vi "TCE_SaveConfiguration.vi"(0 "input cluster":T1={"Core"={"Current VI Reference"=refnum, "Close Panel on Exit?"=FALSE}, "Image Out"="img_0", "State"=0, "Points"={"Top Left"={"X"=54.0, "Y"=69.0}, "Top Right"={"X"=409.0, "Y"=62.0}, "Bottom Left"={"X"=58.0, "Y"=302.0}, "Bottom Right"={"X"=413.0, "Y"=295.0}, "x space 2"=0.2666666805744171, "y space 2"=15.533334, "x_space"=15.434783, "y_space"=-0.3043478, "Pixels"=array384x21[8064 elements], "Fixpoint"={"X"=460.0, "Y"=26.0}}, "img_array"=["img_0", "img_1", "img_2", "img_3", "img_4", "img_5", "img_6", "img_7", "img_8", "img_9", "img_10", "img_11", "img_12", "img_13", "img_14", "img_15", "img_16", "img_17", "img_18", "img_19", "img_20", "img_21", "img_22", "img_23", "img_24", "img_25", "img_26", "img_27", "img_28", "img_29", "img_30", "img_31", "img_32", "img_33", "img_34", "img_35", "img_36", "img_37", "img_38", "img_39", "img_40", "img_41", "img_42", "img_43", "img_44", "img_45", "img_46", "img_47", "img_48", "img_49", "img_50", "img_51", "img_52", "img_53", "img_54", "img_55", "img_56", "img_57", "img_58", "img_59", "img_60", "img_61", "img_62", "img_63", "img_64", "img_65", "img_66", "img_67", "img_68", "img_69", "img_70", "img_71", "img_72", "img_73", "img_74", "img_75", "img_76", "img_77", "img_78", "img_79", "img_80", "img_81", "img_82", "img_83", "img_84", "img_85", "img_86", "img_87", "img_88", "img_89", "img_90", "img_91", "img_92", "img_93", "img_94", "img_95", "img_96", "img_97", "img_98", "img_99", "img_100", "img_101", "img_102", "img_103", "img_104", "img_105", "img_106", "img_107", "img_108", "img_109", "img_110", "img_111", "img_112", "img_113", "img_114", "img_115", "img_116", "img_117", "img_118", "img_119", "img_120", "img_121", "img_122", "img_123", "img_124", "img_125", "img_126", "img_127", "img_128", "img_129", "img_130", "img_131", "img_132", "img_133", "img_134", "img_135", "img_136", "img_137", "img_138", "img_139", "img_140", "img_141", "img_142", "img_143", "img_144", "img_145", "img_146", "img_147", "img_148", "img_149", "img_150", "img_151", "img_152", "img_153", "img_154", "img_155", "img_156", "img_157", "img_158", "img_159", "img_160", "img_161", "img_162", "img_163", "img_164", "img_165", "img_166", "img_167", "img_168", "img_169", "img_170", "img_171", "img_172", "img_173", "img_174", "img_175", "img_176", "img_177", "img_178", "img_179", "img_180", "img_181", "img_182", "img_183", "img_184", "img_185", "img_186", "img_187", "img_188", "img_189", "img_190", "img_191", "img_192", "img_193", "img_194", "img_195", "img_196", "img_197", "img_198", "img_199", "img_200", "img_201", "img_202", "img_203", "img_204", "img_205", "img_206", "img_207", "img_208", "img_209", "img_210", "img_211", "img_212", "img_213", "img_214", "img_215", "img_216", "img_217", "img_218", "img_219", "img_220", "img_221", "img_222", "img_223", "img_224", "img_225", "img_226", "img_227", "img_228", "img_229", "img_230", "img_231", "img_232", "img_233", "img_234", "img_235", "img_236", "img_237", "img_238", "img_239", "img_240", "img_241", "img_242", "img_243", "img_244", "img_245", "img_246", "img_247", "img_248", "img_249", "img_250", "img_251", "img_252", "img_253"], "Temps"=[], "Temps_Array"=[], "Scan Area"=3.0, "Fixpoint Area"=5.0, "Config"={"Freezing"={"Cutoff"=1.0, "EndIndex"=253}}, "PCR Size"=0, "ImageCount"=253, "ShowGradient"=FALSE} {"Points"."Bottom Right"."Y" format="%.2f"; "Points"."Bottom Right"."X" format="%.2f"; "Points"."Top Left"."Y" format="%.2f"; "Points"."Top Left"."X" format="%.2f"; "Points"."Top Right"."Y" format="%.2f"; "Points"."Top Right"."X" format="%.2f"; "Points"."Bottom Left"."Y" format="%.2f"; "Points"."Bottom Left"."X" format="%.2f"; "Points"."Fixpoint"."Y" format="%.2f"; "Points"."Fixpoint"."X" format="%.2f"}, 1 "Temps":dbl[][](graph)=array384x452[173568 elements], 2 "FreezeTemps":dbl[](array[numeric])=[0.0, 0.0, -9.08812883, 0.0, 0.0, 0.0, 0.0, 0.0, 0.0, 0.0, -9.0747955, -11.51009704, 0.0, 0.0, 0.0, 0.0, 0.0, 0.0, 0.0, 0.0, -6.15635948, 0.0, 0.0, 0.0, 0.0, 0.0, 0.0, -8.47241455, 0.0, 0.0, 0.0, 0.0, -8.26812883, -8.60193836, 0.0, -9.01717645, -9.10955741, -2.30476451, -7.81329159, 0.0, 0.0, -8.8147955, 0.0, 0.0, 0.0, 0.0, 0.0, 0.0, 0.0, 0.0, 0.0, -9.36717645, 0.0, -9.36908121, 0.0, 0.0, 0.0, 0.0, 0.0, -8.96765264, -8.71336693, -8.60431931, 0.0, 0.0, -1.50423713, -1.7488225, -1.82501297, -2.09757047, -2.22863306, -2.2188225, 0.0, -2.1609003, 0.0, -1.86328475, -1.81614189, -1.89328125, -1.82470982, -1.57120345, -1.20787012, -1.03518951, -1.55387115, -1.77453678, -1.94371688, -2.22423713, -2.38757047, -2.36852285, -2.20847878, -2.22471332, -2.0088225, -1.91804315, -1.87381212, -1.93545469, -1.78994791, -1.52739393, -1.45354993, -1.04995142, -1.4709003, -1.6835844, -2.11280856, -2.43614189, -2.38929869, -2.51185618, -2.31705021, -2.47947523, -2.36804666, -2.14804315, -1.88280856, -1.96137999, -1.77053782, -1.76196639, -1.25990735, -1.14233237, 0.0, -1.58757047, -1.94804315, -2.22244258, -2.43709428, -2.38705021, -2.23024468, 0.0, -2.24120345, -2.14376094, -1.79800259, -1.91768067, -1.66929869, -1.65185618, -1.53434734, -1.14328475, -1.20501297, -1.52263202, -1.9575264, -2.0127645, -2.13446292, -2.36709428, -2.51661809, -2.37196639, 0.0, -2.08196639, -2.16865453, -1.73705021, -1.65120345, -1.6962521, -1.4535844, 0.0, -1.21116897, -1.55501297, 0.0, -2.26709428, -2.19786373, -2.44376094, -2.59137999, -2.45025107, -2.16783564, -2.18162766, -2.11285974, -1.98047879, -1.83143117, -1.77815687, -1.49328475, -1.24185268, 0.0, -1.42137999, -1.92137649, -1.96990735, -2.34423713, -2.35518951, -2.38137999, -2.2756657, -2.28484501, -2.3200026, -2.09673946, -1.74995142, -1.61423713, -1.51834631, -1.58769184, 0.0, -1.09960692, -1.67008311, -1.95280856, -2.35280856, -2.19895497, -2.02929869, -1.78263202, -1.86215583, -2.1627645, -2.32423713, -1.99800259, -1.92185618, -1.58787012, -1.45501297, -1.53008311, -1.52640707, 0.0, -1.41280856, -1.84215583, -2.28023365, -2.2609038, -1.86042761, -1.70419307, -2.20995142, -2.3656657, -2.26354993, -2.07019909, -1.83895497, -1.72137999, -1.54133592, -1.51137999, -1.35053782, 0.0, -1.2335844, -1.94137999, -1.8975264, -2.1035844, -2.03167964, -2.15943116, -2.34471332, -2.29990735, -2.12895497, -2.06609783, -1.88596536, -1.86466926, -1.7714902, -1.4775264, -1.26720448, -1.16069278, -1.60190736, -1.88638957, -2.02434734, -2.20126039, -2.29736192, -1.99453678, -2.17905022, -2.21376094, -2.07895497, -2.02817834, -2.07815687, -1.94878802, -1.70072726, -1.31644155, -1.39952641, -1.01640707, -1.33196639, -1.84294025, -2.00389263, -2.13272605, -2.2600026, -2.16627358, -2.23627358, -2.24722596, -2.17722596, -2.15627358, -2.0156657, -1.84021659, -1.70589108, -1.45593088, -1.02232887, 0.0, -1.26947523, -1.78722596, -1.9814902, -2.06177367, -2.32285974, -2.38143117, -2.37638957, -2.32734195, -2.21958544, -2.21436882, -2.06021659, -1.78280506, -1.57804666, -1.47137649, -0.97899904, -0.86054899, -1.07878802, -1.3762521, -1.43800259, -1.76899553, -2.03190736, -2.14831183, -2.02518951, -2.25095498, -1.86596536, -1.95470982, -1.87389263, -1.75829433, -1.53614189, -1.29613839, -1.0053212, 0.0, -1.0400728, -1.33674977, -1.58116897, -1.85129748, -1.9600026, -1.82851934, -2.00115147, -2.20809784, -2.03143117, -1.68310821, -1.57514545, -1.60847878, -1.40995142, -1.40874822, 0.0, -0.92593335, -1.13212383, -0.93518951, -1.84118603, -1.49995142, -1.93578708, -1.8407842, -2.09333593, -1.95783564, -2.05857403, -1.96928127, -2.00268896, -1.82054899, -1.65556332, -1.02674977, -1.34640954, -0.3449387, -0.98508713, -0.93307374, -1.45984993, -1.35714546, -1.50381212, -1.32995142, -1.75023365, -1.58636727, -1.78810625, -1.40042761, -1.8052407, -1.69762165, -1.45878802, -0.87865453, -1.00795467, -0.29116897, -1.1165157, -1.05545469, -1.57763006, -1.12294025, -1.50688326, -1.39067528, -1.25328125, -1.65212204, -1.71883978, -1.69748796, -1.71526146, -1.46428832, -1.38116897, -1.05889755, -1.07318327, -0.27714546, -0.77333593, -0.86878802, -1.24763006, -1.20413474, -0.88768067, -1.12126039, -1.23177367, -1.29413474, -1.30573765, -1.18816803, -1.13190736, -0.72913073, -1.02509752, -0.25804666, -0.07781814, -0.83402612, -1.28878802, -1.82334435, -1.44545469, -1.83603951, -1.15947172, -1.9512785, -1.58047879, -1.42353243, -1.46619308, -1.35994791, -1.64260002, -1.38115147, -1.34531089, -1.4581186, -0.9295966], 3 "MeltTemps":dbl[](array[numeric])=[0.0, 0.0, -0.4342733, 0.0, 0.0, 0.0, 0.0, 0.0, 0.0, 0.0, -0.62680341, -0.51224316, 0.0, 0.0, 0.0, 0.0, 0.0, 0.0, 0.0, 0.0, -0.22420383, 0.0, 0.0, 0.0, 0.0, 0.0, 0.0, -0.49056915, 0.0, 0.0, 0.0, 0.0, -0.43469229, -0.33454438, 0.0, -0.71724972, -0.58354536, 0.3398814, 0.1094774, 0.0, 0.0, -0.21594961, 0.0, 0.0, 0.0, 0.0, 0.0, 0.0, 0.0, 0.0, 0.0, 0.08689311, 0.0, 0.19815221, 0.0, 0.0, 0.0, 0.0, 0.0, 0.21934158, -0.38069337, 0.32423894, 0.0, 0.0, -0.27254066, -0.24847196, -0.2403621, -0.27746832, -0.29275768, -0.38444542, 0.0, -0.31968351, 0.0, -0.28131448, -0.26609101, -0.25751958, -0.17132911, -0.15323387, 0.08177022, -0.18364134, -0.28847196, -0.1565672, -0.20894815, -0.27083829, -0.37940972, -0.35223116, -0.32369543, -0.32889782, -0.28223023, -0.17524899, -0.11682637, -0.14893353, -0.05513863, -0.00223023, -0.01179305, -0.07982523, -0.21275768, -0.09561482, -0.19873113, -0.35111209, -0.39444542, -0.43635018, -0.35635018, -0.38635018, -0.33682637, -0.2253978, -0.17704339, -0.07323387, -0.1050883, -0.08607876, 0.03129403, -0.1065672, 0.0, -0.03799577, -0.14968351, -0.2506221, -0.38349304, -0.39966972, -0.36275768, 0.0, -0.36030142, -0.18942434, -0.14942434, -0.14492161, -0.07179305, -0.03513863, 0.00174506, -0.15371006, -0.10561482, 0.03468434, -0.20842071, -0.22461118, -0.30301685, -0.34798114, -0.34464781, -0.33083829, 0.0, -0.24417162, -0.20321924, -0.12918216, -0.09323387, 0.03205549, 0.06700831, 0.0, -0.09561482, -0.04858474, 0.0, -0.26492161, -0.36746832, -0.38301685, -0.440781, -0.40873113, -0.23635018, -0.23889782, -0.15649529, -0.14432215, -0.11587399, -0.08908405, 0.04967453, -0.18775359, 0.0, 0.09248042, -0.05799577, -0.19751958, -0.30274305, -0.32443162, -0.33226686, -0.31988591, -0.285124, -0.27744767, -0.22459052, -0.10702876, 0.01105185, 0.01152804, 0.05174506, 0.0, 0.15255573, 0.08318743, -0.09037673, -0.30369543, -0.25466244, -0.2018053, -0.13635018, -0.16323387, -0.30704339, -0.30127878, -0.19275768, -0.12777875, 0.01581375, 0.12581375, 0.10555458, -0.08836967, 0.0, 0.11295661, -0.09847196, -0.2530189, -0.26942434, -0.11254066, -0.18444542, -0.29459052, -0.37098881, -0.27080258, -0.20682637, -0.04228149, -0.05704339, 0.06200423, 0.04841172, -0.05268576, 0.0, 0.22093907, -0.04560257, -0.15275768, -0.22322162, -0.23396923, -0.26842071, -0.34206447, -0.32080166, -0.22442026, -0.18799577, -0.09037673, -0.08561482, -0.02037673, 0.07373196, -0.11965835, 0.1401498, 0.16841172, 0.02412601, -0.08444542, -0.11444542, -0.22982862, -0.21349304, -0.1660191, -0.21792386, -0.20349304, -0.12730256, -0.13730256, -0.01682637, 0.05390899, 0.17581375, -0.14323387, 0.14126887, 0.22628994, 0.06031649, 0.00725695, -0.01063589, -0.10887624, -0.15607876, -0.20604068, -0.19492161, -0.10111209, -0.12063589, -0.05199541, 0.03745934, 0.15533756, 0.19570097, -0.00132911, 0.0, 0.28771851, 0.14364982, -0.01158828, -0.05175497, -0.05206447, -0.11730256, -0.14173338, -0.1453978, -0.10275768, -0.09396923, 0.00412601, 0.02962327, 0.18986546, 0.21581375, 0.07087482, 0.30936411, 0.48046529, 0.2598403, 0.08248042, 0.05914708, -0.00396923, -0.07920732, -0.06323387, -0.05920732, -0.0018053, 0.02105185, 0.03446049, 0.09200423, 0.24510355, 0.33200423, 0.18771851, 0.0, 0.56636525, 0.32962327, 0.27698315, 0.14603077, 0.1246022, 0.01820933, 0.05867089, 0.03222125, 0.1046022, 0.07152804, 0.12867089, 0.12438518, 0.32057566, 0.3498403, 0.0, 0.43650696, 0.67317363, 0.44065096, 0.23826662, 0.18189145, 0.19603077, 0.17348313, 0.0746022, 0.20064757, 0.17079268, 0.13064757, 0.15064757, 0.27555458, 0.34793553, 0.55856053, 0.23729265, 0.64507839, 0.82271123, 0.65141767, 0.49454726, 0.44731763, 0.34175885, 0.30364982, 0.29207614, 0.34630219, 0.28586408, 0.27284624, 0.31963552, 0.41555458, 0.50350811, 0.67427481, 0.32126887, 0.90962327, 0.72110218, 0.63207954, 0.5249117, 0.55724232, 0.35588906, 0.39296886, 0.37112716, 0.39364982, 0.35534981, 0.34318743, 0.48317363, 0.56392124, 0.51684144, 0.78126887, 0.44031649, 0.93438518, 0.8598403, 0.76160335, 0.7246022, 0.61996357, 0.6134328, 0.62317363, 0.6101498, 0.59776884, 0.60174506, 0.65237005, 0.74808434, 0.75538882, 0.77603077, 0.9334328, 0.89628994, 0.46919834, 0.46582838, 0.25269744, 0.32868314, 0.35493328, 0.43676613, 0.22793553, 0.35017138, 0.3305879, 0.41079268, 0.29200423, 0.3396379, 0.38106647, 0.59009947, 0.53628994, 0.55200423], 4 "FrozenFraction":dbl[](array[numeric])=[-0.058823529411764705, -0.058823529411764705, 0.7647058823529411, -0.058823529411764705, -0.058823529411764705, -0.058823529411764705, -0.058823529411764705, -0.058823529411764705, -0.058823529411764705, -0.058823529411764705, 0.7058823529411765, 1.0, -0.058823529411764705, -0.058823529411764705, -0.058823529411764705, -0.058823529411764705, -0.058823529411764705, -0.058823529411764705, -0.058823529411764705, -0.058823529411764705, 0.11764705882352941, -0.058823529411764705, -0.058823529411764705, -0.058823529411764705, -0.058823529411764705, -0.058823529411764705, -0.058823529411764705, 0.29411764705882354, -0.058823529411764705, -0.058823529411764705, -0.058823529411764705, -0.058823529411764705, 0.23529411764705882, 0.35294117647058826, -0.058823529411764705, 0.6470588235294118, 0.8235294117647058, 0.058823529411764705, 0.17647058823529413, -0.058823529411764705, -0.058823529411764705, 0.5294117647058824, -0.058823529411764705, -0.058823529411764705, -0.058823529411764705, -0.058823529411764705, -0.058823529411764705, -0.058823529411764705, -0.058823529411764705, -0.058823529411764705, -0.058823529411764705, 0.8823529411764706, -0.058823529411764705, 0.9411764705882353, -0.058823529411764705, -0.058823529411764705, -0.058823529411764705, -0.058823529411764705, -0.058823529411764705, 0.5882352941176471, 0.47058823529411764, 0.4117647058823529, -0.058823529411764705, -0.058823529411764705, 0.14864864864864866, 0.32432432432432434, 0.43243243243243246, 0.6351351351351351, 0.7972972972972973, 0.7432432432432432, -0.013513513513513514, 0.7027027027027027, -0.013513513513513514, 0.44594594594594594, 0.40540540540540543, 0.4864864864864865, 0.4189189189189189, 0.21621621621621623, 0.08108108108108109, 0.013513513513513514, 0.20270270270270271, 0.36486486486486486, 0.5405405405405406, 0.7702702702702703, 0.918918918918919, 0.8783783783783784, 0.7297297297297297, 0.7837837837837838, 0.5945945945945946, 0.5135135135135135, 0.4594594594594595, 0.527027027027027, 0.3783783783783784, 0.17567567567567569, 0.10810810810810811, 0.02702702702702703, 0.13513513513513514, 0.28378378378378377, 0.6486486486486487, 0.9459459459459459, 0.9324324324324325, 0.9864864864864865, 0.8378378378378378, 0.972972972972973, 0.8648648648648649, 0.6891891891891891, 0.47297297297297297, 0.581081081081081, 0.35135135135135137, 0.33783783783783783, 0.0945945945945946, 0.04054054054054054, -0.013513513513513514, 0.22972972972972974, 0.5540540540540541, 0.7567567567567568, 0.9594594594594594, 0.9054054054054054, 0.8108108108108109, -0.013513513513513514, 0.8243243243243243, 0.6756756756756757, 0.3918918918918919, 0.5, 0.2702702702702703, 0.25675675675675674, 0.1891891891891892, 0.05405405405405406, 0.06756756756756757, 0.16216216216216217, 0.5675675675675675, 0.6081081081081081, 0.6621621621621622, 0.8513513513513513, 1.0, 0.8918918918918919, -0.013513513513513514, 0.6216216216216216, 0.7162162162162162, 0.3108108108108108, 0.24324324324324326, 0.2972972972972973, 0.12162162162162163, -0.013513513513513514, 0.02666666666666667, 0.22666666666666666, -0.013333333333333334, 0.8, 0.7333333333333333, 0.9733333333333334, 1.0, 0.9866666666666667, 0.7066666666666667, 0.72, 0.6533333333333333, 0.5466666666666666, 0.37333333333333335, 0.3466666666666667, 0.14666666666666667, 0.05333333333333334, -0.013333333333333334, 0.10666666666666667, 0.48, 0.5333333333333333, 0.8933333333333333, 0.9333333333333333, 0.96, 0.8133333333333334, 0.84, 0.8666666666666667, 0.6266666666666667, 0.32, 0.26666666666666666, 0.17333333333333334, 0.24, -0.013333333333333334, 0.013333333333333334, 0.28, 0.52, 0.92, 0.7466666666666667, 0.5733333333333334, 0.36, 0.4266666666666667, 0.6933333333333334, 0.88, 0.56, 0.49333333333333335, 0.25333333333333335, 0.12, 0.2, 0.18666666666666668, -0.013333333333333334, 0.09333333333333334, 0.4, 0.8266666666666667, 0.7733333333333333, 0.41333333333333333, 0.29333333333333333, 0.76, 0.9466666666666667, 0.7866666666666666, 0.6133333333333333, 0.38666666666666666, 0.30666666666666664, 0.21333333333333335, 0.16, 0.08, -0.013333333333333334, 0.04, 0.5066666666666667, 0.4666666666666667, 0.64, 0.5866666666666667, 0.68, 0.9066666666666666, 0.8533333333333334, 0.6666666666666666, 0.6, 0.4533333333333333, 0.44, 0.3333333333333333, 0.13333333333333333, 0.06666666666666667, 0.1038961038961039, 0.3246753246753247, 0.5194805194805194, 0.6363636363636364, 0.8311688311688312, 0.948051948051948, 0.5844155844155844, 0.8181818181818182, 0.8571428571428571, 0.7402597402597403, 0.6623376623376623, 0.7272727272727273, 0.5324675324675324, 0.36363636363636365, 0.14285714285714285, 0.19480519480519481, 0.05194805194805195, 0.15584415584415584, 0.4675324675324675, 0.6103896103896104, 0.7532467532467533, 0.935064935064935, 0.7922077922077922, 0.8961038961038961, 0.9090909090909091, 0.8051948051948052, 0.7792207792207793, 0.6233766233766234, 0.45454545454545453, 0.37662337662337664, 0.24675324675324675, 0.06493506493506493, -0.012987012987012988, 0.11688311688311688, 0.42857142857142855, 0.5714285714285714, 0.7142857142857143, 0.961038961038961, 1.0, 0.987012987012987, 0.974025974025974, 0.8831168831168831, 0.8701298701298701, 0.7012987012987013, 0.4155844155844156, 0.2987012987012987, 0.2597402597402597, 0.025974025974025976, 0.012987012987012988, 0.09090909090909091, 0.18181818181818182, 0.23376623376623376, 0.4025974025974026, 0.6883116883116883, 0.7662337662337663, 0.6493506493506493, 0.922077922077922, 0.4935064935064935, 0.5454545454545454, 0.5064935064935064, 0.38961038961038963, 0.2727272727272727, 0.12987012987012986, 0.03896103896103896, -0.012987012987012988, 0.07792207792207792, 0.16883116883116883, 0.3116883116883117, 0.4805194805194805, 0.5584415584415584, 0.44155844155844154, 0.5974025974025974, 0.8441558441558441, 0.6753246753246753, 0.35064935064935066, 0.2857142857142857, 0.33766233766233766, 0.22077922077922077, 0.2077922077922078, -0.012987012987012988, 0.15, 0.3375, 0.1875, 0.9125, 0.6625, 0.925, 0.9, 1.0, 0.95, 0.9875, 0.9625, 0.975, 0.8625, 0.7625, 0.2375, 0.4875, 0.0625, 0.2, 0.175, 0.625, 0.5, 0.675, 0.4625, 0.825, 0.725, 0.8375, 0.5625, 0.85, 0.7875, 0.6125, 0.125, 0.2125, 0.05, 0.2875, 0.25, 0.7, 0.3125, 0.6875, 0.55, 0.4125, 0.75, 0.8125, 0.775, 0.8, 0.6375, 0.5375, 0.2625, 0.275, 0.0375, 0.0875, 0.1125, 0.4, 0.375, 0.1375, 0.3, 0.3875, 0.4375, 0.45, 0.3625, 0.325, 0.075, 0.225, 0.025, 0.0125, 0.1, 0.425, 0.875, 0.5875, 0.8875, 0.35, 0.9375, 0.7125, 0.575, 0.65, 0.5125, 0.7375, 0.525, 0.475, 0.6, 0.1625], 5 "PartitionArray":string[](array[string])=["A, MQ filtered", "A, MQ filtered", "A, MQ filtered", "A, MQ filtered", "A, MQ filtered", "A, MQ filtered", "A, MQ filtered", "A, MQ filtered", "A, MQ filtered", "A, MQ filtered", "A, MQ filtered", "A, MQ filtered", "A, MQ filtered", "A, MQ filtered", "A, MQ filtered", "A, MQ filtered", "A, MQ filtered", "A, MQ filtered", "A, MQ filtered", "A, MQ filtered", "A, MQ filtered", "A, MQ filtered", "A, MQ filtered", "A, MQ filtered", "A, MQ filtered", "A, MQ filtered", "A, MQ filtered", "A, MQ filtered", "A, MQ filtered", "A, MQ filtered", "A, MQ filtered", "A, MQ filtered", "A, MQ filtered", "A, MQ filtered", "A, MQ filtered", "A, MQ filtered", "A, MQ filtered", "A, MQ filtered", "A, MQ filtered", "A, MQ filtered", "A, MQ filtered", "A, MQ filtered", "A, MQ filtered", "A, MQ filtered", "A, MQ filtered", "A, MQ filtered", "A, MQ filtered", "A, MQ filtered", "A, MQ filtered", "A, MQ filtered", "A, MQ filtered", "A, MQ filtered", "A, MQ filtered", "A, MQ filtered", "A, MQ filtered", "A, MQ filtered", "A, MQ filtered", "A, MQ filtered", "A, MQ filtered", "A, MQ filtered", "A, MQ filtered", "A, MQ filtered", "A, MQ filtered", "A, MQ filtered", "B, 220628_Psyringae_L_8days_c1", "B, 220628_Psyringae_L_8days_c1", "B, 220628_Psyringae_L_8days_c1", "B, 220628_Psyringae_L_8days_c1", "B, 220628_Psyringae_L_8days_c1", "B, 220628_Psyringae_L_8days_c1", "B, 220628_Psyringae_L_8days_c1", "B, 220628_Psyringae_L_8days_c1", "B, 220628_Psyringae_L_8days_c1", "B, 220628_Psyringae_L_8days_c1", "B, 220628_Psyringae_L_8days_c1", "B, 220628_Psyringae_L_8days_c1", "B, 220628_Psyringae_L_8days_c1", "B, 220628_Psyringae_L_8days_c1", "B, 220628_Psyringae_L_8days_c1", "B, 220628_Psyringae_L_8days_c1", "B, 220628_Psyringae_L_8days_c1", "B, 220628_Psyringae_L_8days_c1", "B, 220628_Psyringae_L_8days_c1", "B, 220628_Psyringae_L_8days_c1", "B, 220628_Psyringae_L_8days_c1", "B, 220628_Psyringae_L_8days_c1", "B, 220628_Psyringae_L_8days_c1", "B, 220628_Psyringae_L_8days_c1", "B, 220628_Psyringae_L_8days_c1", "B, 220628_Psyringae_L_8days_c1", "B, 220628_Psyringae_L_8days_c1", "B, 220628_Psyringae_L_8days_c1", "B, 220628_Psyringae_L_8days_c1", "B, 220628_Psyringae_L_8days_c1", "B, 220628_Psyringae_L_8days_c1", "B, 220628_Psyringae_L_8days_c1", "B, 220628_Psyringae_L_8days_c1", "B, 220628_Psyringae_L_8days_c1", "B, 220628_Psyringae_L_8days_c1", "B, 220628_Psyringae_L_8days_c1", "B, 220628_Psyringae_L_8days_c1", "B, 220628_Psyringae_L_8days_c1", "B, 220628_Psyringae_L_8days_c1", "B, 220628_Psyringae_L_8days_c1", "B, 220628_Psyringae_L_8days_c1", "B, 220628_Psyringae_L_8days_c1", "B, 220628_Psyringae_L_8days_c1", "B, 220628_Psyringae_L_8days_c1", "B, 220628_Psyringae_L_8days_c1", "B, 220628_Psyringae_L_8days_c1", "B, 220628_Psyringae_L_8days_c1", "B, 220628_Psyringae_L_8days_c1", "B, 220628_Psyringae_L_8days_c1", "B, 220628_Psyringae_L_8days_c1", "B, 220628_Psyringae_L_8days_c1", "B, 220628_Psyringae_L_8days_c1", "B, 220628_Psyringae_L_8days_c1", "B, 220628_Psyringae_L_8days_c1", "B, 220628_Psyringae_L_8days_c1", "B, 220628_Psyringae_L_8days_c1", "B, 220628_Psyringae_L_8days_c1", "B, 220628_Psyringae_L_8days_c1", "B, 220628_Psyringae_L_8days_c1", "B, 220628_Psyringae_L_8days_c1", "B, 220628_Psyringae_L_8days_c1", "B, 220628_Psyringae_L_8days_c1", "B, 220628_Psyringae_L_8days_c1", "B, 220628_Psyringae_L_8days_c1", "B, 220628_Psyringae_L_8days_c1", "B, 220628_Psyringae_L_8days_c1", "B, 220628_Psyringae_L_8days_c1", "B, 220628_Psyringae_L_8days_c1", "B, 220628_Psyringae_L_8days_c1", "B, 220628_Psyringae_L_8days_c1", "B, 220628_Psyringae_L_8days_c1", "B, 220628_Psyringae_L_8days_c1", "B, 220628_Psyringae_L_8days_c1", "B, 220628_Psyringae_L_8days_c1", "B, 220628_Psyringae_L_8days_c1", "B, 220628_Psyringae_L_8days_c1", "B, 220628_Psyringae_L_8days_c1", "B, 220628_Psyringae_L_8days_c1", "B, 220628_Psyringae_L_8days_c1", "B, 220628_Psyringae_L_8days_c1", "C, 220628_Psyringae_L_8days_c1_10fold_dil", "C, 220628_Psyringae_L_8days_c1_10fold_dil", "C, 220628_Psyringae_L_8days_c1_10fold_dil", "C, 220628_Psyringae_L_8days_c1_10fold_dil", "C, 220628_Psyringae_L_8days_c1_10fold_dil", "C, 220628_Psyringae_L_8days_c1_10fold_dil", "C, 220628_Psyringae_L_8days_c1_10fold_dil", "C, 220628_Psyringae_L_8days_c1_10fold_dil", "C, 220628_Psyringae_L_8days_c1_10fold_dil", "C, 220628_Psyringae_L_8days_c1_10fold_dil", "C, 220628_Psyringae_L_8days_c1_10fold_dil", "C, 220628_Psyringae_L_8days_c1_10fold_dil", "C, 220628_Psyringae_L_8days_c1_10fold_dil", "C, 220628_Psyringae_L_8days_c1_10fold_dil", "C, 220628_Psyringae_L_8days_c1_10fold_dil", "C, 220628_Psyringae_L_8days_c1_10fold_dil", "C, 220628_Psyringae_L_8days_c1_10fold_dil", "C, 220628_Psyringae_L_8days_c1_10fold_dil", "C, 220628_Psyringae_L_8days_c1_10fold_dil", "C, 220628_Psyringae_L_8days_c1_10fold_dil", "C, 220628_Psyringae_L_8days_c1_10fold_dil", "C, 220628_Psyringae_L_8days_c1_10fold_dil", "C, 220628_Psyringae_L_8days_c1_10fold_dil", "C, 220628_Psyringae_L_8days_c1_10fold_dil", "C, 220628_Psyringae_L_8days_c1_10fold_dil", "C, 220628_Psyringae_L_8days_c1_10fold_dil", "C, 220628_Psyringae_L_8days_c1_10fold_dil", "C, 220628_Psyringae_L_8days_c1_10fold_dil", "C, 220628_Psyringae_L_8days_c1_10fold_dil", "C, 220628_Psyringae_L_8days_c1_10fold_dil", "C, 220628_Psyringae_L_8days_c1_10fold_dil", "C, 220628_Psyringae_L_8days_c1_10fold_dil", "C, 220628_Psyringae_L_8days_c1_10fold_dil", "C, 220628_Psyringae_L_8days_c1_10fold_dil", "C, 220628_Psyringae_L_8days_c1_10fold_dil", "C, 220628_Psyringae_L_8days_c1_10fold_dil", "C, 220628_Psyringae_L_8days_c1_10fold_dil", "C, 220628_Psyringae_L_8days_c1_10fold_dil", "C, 220628_Psyringae_L_8days_c1_10fold_dil", "C, 220628_Psyringae_L_8days_c1_10fold_dil", "C, 220628_Psyringae_L_8days_c1_10fold_dil", "C, 220628_Psyringae_L_8days_c1_10fold_dil", "C, 220628_Psyringae_L_8days_c1_10fold_dil", "C, 220628_Psyringae_L_8days_c1_10fold_dil", "C, 220628_Psyringae_L_8days_c1_10fold_dil", "C, 220628_Psyringae_L_8days_c1_10fold_dil", "C, 220628_Psyringae_L_8days_c1_10fold_dil", "C, 220628_Psyringae_L_8days_c1_10fold_dil", "C, 220628_Psyringae_L_8days_c1_10fold_dil", "C, 220628_Psyringae_L_8days_c1_10fold_dil", "C, 220628_Psyringae_L_8days_c1_10fold_dil", "C, 220628_Psyringae_L_8days_c1_10fold_dil", "C, 220628_Psyringae_L_8days_c1_10fold_dil", "C, 220628_Psyringae_L_8days_c1_10fold_dil", "C, 220628_Psyringae_L_8days_c1_10fold_dil", "C, 220628_Psyringae_L_8days_c1_10fold_dil", "C, 220628_Psyringae_L_8days_c1_10fold_dil", "C, 220628_Psyringae_L_8days_c1_10fold_dil", "C, 220628_Psyringae_L_8days_c1_10fold_dil", "C, 220628_Psyringae_L_8days_c1_10fold_dil", "C, 220628_Psyringae_L_8days_c1_10fold_dil", "C, 220628_Psyringae_L_8days_c1_10fold_dil", "C, 220628_Psyringae_L_8days_c1_10fold_dil", "C, 220628_Psyringae_L_8days_c1_10fold_dil", "C, 220628_Psyringae_L_8days_c1_10fold_dil", "C, 220628_Psyringae_L_8days_c1_10fold_dil", "C, 220628_Psyringae_L_8days_c1_10fold_dil", "C, 220628_Psyringae_L_8days_c1_10fold_dil", "C, 220628_Psyringae_L_8days_c1_10fold_dil", "C, 220628_Psyringae_L_8days_c1_10fold_dil", "C, 220628_Psyringae_L_8days_c1_10fold_dil", "C, 220628_Psyringae_L_8days_c1_10fold_dil", "C, 220628_Psyringae_L_8days_c1_10fold_dil", "C, 220628_Psyringae_L_8days_c1_10fold_dil", "C, 220628_Psyringae_L_8days_c1_10fold_dil", "C, 220628_Psyringae_L_8days_c1_10fold_dil", "C, 220628_Psyringae_L_8days_c1_10fold_dil", "C, 220628_Psyringae_L_8days_c1_10fold_dil", "C, 220628_Psyringae_L_8days_c1_10fold_dil", "C, 220628_Psyringae_L_8days_c1_10fold_dil", "D, 220628_Psyringae_L_8days_c1_100fold_dil", "D, 220628_Psyringae_L_8days_c1_100fold_dil", "D, 220628_Psyringae_L_8days_c1_100fold_dil", "D, 220628_Psyringae_L_8days_c1_100fold_dil", "D, 220628_Psyringae_L_8days_c1_100fold_dil", "D, 220628_Psyringae_L_8days_c1_100fold_dil", "D, 220628_Psyringae_L_8days_c1_100fold_dil", "D, 220628_Psyringae_L_8days_c1_100fold_dil", "D, 220628_Psyringae_L_8days_c1_100fold_dil", "D, 220628_Psyringae_L_8days_c1_100fold_dil", "D, 220628_Psyringae_L_8days_c1_100fold_dil", "D, 220628_Psyringae_L_8days_c1_100fold_dil", "D, 220628_Psyringae_L_8days_c1_100fold_dil", "D, 220628_Psyringae_L_8days_c1_100fold_dil", "D, 220628_Psyringae_L_8days_c1_100fold_dil", "D, 220628_Psyringae_L_8days_c1_100fold_dil", "D, 220628_Psyringae_L_8days_c1_100fold_dil", "D, 220628_Psyringae_L_8days_c1_100fold_dil", "D, 220628_Psyringae_L_8days_c1_100fold_dil", "D, 220628_Psyringae_L_8days_c1_100fold_dil", "D, 220628_Psyringae_L_8days_c1_100fold_dil", "D, 220628_Psyringae_L_8days_c1_100fold_dil", "D, 220628_Psyringae_L_8days_c1_100fold_dil", "D, 220628_Psyringae_L_8days_c1_100fold_dil", "D, 220628_Psyringae_L_8days_c1_100fold_dil", "D, 220628_Psyringae_L_8days_c1_100fold_dil", "D, 220628_Psyringae_L_8days_c1_100fold_dil", "D, 220628_Psyringae_L_8days_c1_100fold_dil", "D, 220628_Psyringae_L_8days_c1_100fold_dil", "D, 220628_Psyringae_L_8days_c1_100fold_dil", "D, 220628_Psyringae_L_8days_c1_100fold_dil", "D, 220628_Psyringae_L_8days_c1_100fold_dil", "D, 220628_Psyringae_L_8days_c1_100fold_dil", "D, 220628_Psyringae_L_8days_c1_100fold_dil", "D, 220628_Psyringae_L_8days_c1_100fold_dil", "D, 220628_Psyringae_L_8days_c1_100fold_dil", "D, 220628_Psyringae_L_8days_c1_100fold_dil", "D, 220628_Psyringae_L_8days_c1_100fold_dil", "D, 220628_Psyringae_L_8days_c1_100fold_dil", "D, 220628_Psyringae_L_8days_c1_100fold_dil", "D, 220628_Psyringae_L_8days_c1_100fold_dil", "D, 220628_Psyringae_L_8days_c1_100fold_dil", "D, 220628_Psyringae_L_8days_c1_100fold_dil", "D, 220628_Psyringae_L_8days_c1_100fold_dil", "D, 220628_Psyringae_L_8days_c1_100fold_dil", "D, 220628_Psyringae_L_8days_c1_100fold_dil", "D, 220628_Psyringae_L_8days_c1_100fold_dil", "D, 220628_Psyringae_L_8days_c1_100fold_dil", "D, 220628_Psyringae_L_8days_c1_100fold_dil", "D, 220628_Psyringae_L_8days_c1_100fold_dil", "D, 220628_Psyringae_L_8days_c1_100fold_dil", "D, 220628_Psyringae_L_8days_c1_100fold_dil", "D, 220628_Psyringae_L_8days_c1_100fold_dil", "D, 220628_Psyringae_L_8days_c1_100fold_dil", "D, 220628_Psyringae_L_8days_c1_100fold_dil", "D, 220628_Psyringae_L_8days_c1_100fold_dil", "D, 220628_Psyringae_L_8days_c1_100fold_dil", "D, 220628_Psyringae_L_8days_c1_100fold_dil", "D, 220628_Psyringae_L_8days_c1_100fold_dil", "D, 220628_Psyringae_L_8days_c1_100fold_dil", "D, 220628_Psyringae_L_8days_c1_100fold_dil", "D, 220628_Psyringae_L_8days_c1_100fold_dil", "D, 220628_Psyringae_L_8days_c1_100fold_dil", "D, 220628_Psyringae_L_8days_c1_100fold_dil", "D, 220628_Psyringae_L_8days_c1_100fold_dil", "D, 220628_Psyringae_L_8days_c1_100fold_dil", "D, 220628_Psyringae_L_8days_c1_100fold_dil", "D, 220628_Psyringae_L_8days_c1_100fold_dil", "D, 220628_Psyringae_L_8days_c1_100fold_dil", "D, 220628_Psyringae_L_8days_c1_100fold_dil", "D, 220628_Psyringae_L_8days_c1_100fold_dil", "D, 220628_Psyringae_L_8days_c1_100fold_dil", "D, 220628_Psyringae_L_8days_c1_100fold_dil", "D, 220628_Psyringae_L_8days_c1_100fold_dil", "D, 220628_Psyringae_L_8days_c1_100fold_dil", "D, 220628_Psyringae_L_8days_c1_100fold_dil", "D, 220628_Psyringae_L_8days_c1_100fold_dil", "D, 220628_Psyringae_L_8days_c1_100fold_dil", "D, 220628_Psyringae_L_8days_c1_100fold_dil", "D, 220628_Psyringae_L_8days_c1_100fold_dil", "E, 220628_Psyringae_L_8days_c1_1000fold_dil", "E, 220628_Psyringae_L_8days_c1_1000fold_dil", "E, 220628_Psyringae_L_8days_c1_1000fold_dil", "E, 220628_Psyringae_L_8days_c1_1000fold_dil", "E, 220628_Psyringae_L_8days_c1_1000fold_dil", "E, 220628_Psyringae_L_8days_c1_1000fold_dil", "E, 220628_Psyringae_L_8days_c1_1000fold_dil", "E, 220628_Psyringae_L_8days_c1_1000fold_dil", "E, 220628_Psyringae_L_8days_c1_1000fold_dil", "E, 220628_Psyringae_L_8days_c1_1000fold_dil", "E, 220628_Psyringae_L_8days_c1_1000fold_dil", "E, 220628_Psyringae_L_8days_c1_1000fold_dil", "E, 220628_Psyringae_L_8days_c1_1000fold_dil", "E, 220628_Psyringae_L_8days_c1_1000fold_dil", "E, 220628_Psyringae_L_8days_c1_1000fold_dil", "E, 220628_Psyringae_L_8days_c1_1000fold_dil", "E, 220628_Psyringae_L_8days_c1_1000fold_dil", "E, 220628_Psyringae_L_8days_c1_1000fold_dil", "E, 220628_Psyringae_L_8days_c1_1000fold_dil", "E, 220628_Psyringae_L_8days_c1_1000fold_dil", "E, 220628_Psyringae_L_8days_c1_1000fold_dil", "E, 220628_Psyringae_L_8days_c1_1000fold_dil", "E, 220628_Psyringae_L_8days_c1_1000fold_dil", "E, 220628_Psyringae_L_8days_c1_1000fold_dil", "E, 220628_Psyringae_L_8days_c1_1000fold_dil", "E, 220628_Psyringae_L_8days_c1_1000fold_dil", "E, 220628_Psyringae_L_8days_c1_1000fold_dil", "E, 220628_Psyringae_L_8days_c1_1000fold_dil", "E, 220628_Psyringae_L_8days_c1_1000fold_dil", "E, 220628_Psyringae_L_8days_c1_1000fold_dil", "E, 220628_Psyringae_L_8days_c1_1000fold_dil", "E, 220628_Psyringae_L_8days_c1_1000fold_dil", "E, 220628_Psyringae_L_8days_c1_1000fold_dil", "E, 220628_Psyringae_L_8days_c1_1000fold_dil", "E, 220628_Psyringae_L_8days_c1_1000fold_dil", "E, 220628_Psyringae_L_8days_c1_1000fold_dil", "E, 220628_Psyringae_L_8days_c1_1000fold_dil", "E, 220628_Psyringae_L_8days_c1_1000fold_dil", "E, 220628_Psyringae_L_8days_c1_1000fold_dil", "E, 220628_Psyringae_L_8days_c1_1000fold_dil", "E, 220628_Psyringae_L_8days_c1_1000fold_dil", "E, 220628_Psyringae_L_8days_c1_1000fold_dil", "E, 220628_Psyringae_L_8days_c1_1000fold_dil", "E, 220628_Psyringae_L_8days_c1_1000fold_dil", "E, 220628_Psyringae_L_8days_c1_1000fold_dil", "E, 220628_Psyringae_L_8days_c1_1000fold_dil", "E, 220628_Psyringae_L_8days_c1_1000fold_dil", "E, 220628_Psyringae_L_8days_c1_1000fold_dil", "E, 220628_Psyringae_L_8days_c1_1000fold_dil", "E, 220628_Psyringae_L_8days_c1_1000fold_dil", "E, 220628_Psyringae_L_8days_c1_1000fold_dil", "E, 220628_Psyringae_L_8days_c1_1000fold_dil", "E, 220628_Psyringae_L_8days_c1_1000fold_dil", "E, 220628_Psyringae_L_8days_c1_1000fold_dil", "E, 220628_Psyringae_L_8days_c1_1000fold_dil", "E, 220628_Psyringae_L_8days_c1_1000fold_dil", "E, 220628_Psyringae_L_8days_c1_1000fold_dil", "E, 220628_Psyringae_L_8days_c1_1000fold_dil", "E, 220628_Psyringae_L_8days_c1_1000fold_dil", "E, 220628_Psyringae_L_8days_c1_1000fold_dil", "E, 220628_Psyringae_L_8days_c1_1000fold_dil", "E, 220628_Psyringae_L_8days_c1_1000fold_dil", "E, 220628_Psyringae_L_8days_c1_1000fold_dil", "E, 220628_Psyringae_L_8days_c1_1000fold_dil", "E, 220628_Psyringae_L_8days_c1_1000fold_dil", "E, 220628_Psyringae_L_8days_c1_1000fold_dil", "E, 220628_Psyringae_L_8days_c1_1000fold_dil", "E, 220628_Psyringae_L_8days_c1_1000fold_dil", "E, 220628_Psyringae_L_8days_c1_1000fold_dil", "E, 220628_Psyringae_L_8days_c1_1000fold_dil", "E, 220628_Psyringae_L_8days_c1_1000fold_dil", "E, 220628_Psyringae_L_8days_c1_1000fold_dil", "E, 220628_Psyringae_L_8days_c1_1000fold_dil", "E, 220628_Psyringae_L_8days_c1_1000fold_dil", "E, 220628_Psyringae_L_8days_c1_1000fold_dil", "E, 220628_Psyringae_L_8days_c1_1000fold_dil", "E, 220628_Psyringae_L_8days_c1_1000fold_dil", "E, 220628_Psyringae_L_8days_c1_1000fold_dil", "E, 220628_Psyringae_L_8days_c1_1000fold_dil", "E, 220628_Psyringae_L_8days_c1_1000fold_dil"], 7 "Offsets":dbl[](array[numeric])=[-0.90334019, -0.9161796, -0.80332393, -0.7834149, -0.82643058, -0.6685973, -0.74360948, -0.72258592, -0.70246108, -0.75416764, -0.73348982, -0.761681, -0.83858132, -0.76590043, -0.84169212, -0.79199164, -0.8463463, -0.76526398, -0.83821629, -0.91694116, -0.90690966, -0.68424699, -0.69370753, -0.71219233, -0.70905376, -0.67816346, -0.67457819, -0.62920248, -0.72726665, -0.69636261, -0.75405438, -0.67261546, -0.62911746, -0.69727554, -0.69403039, -0.74297488, -0.72961984, -0.73014797, -0.63921766, -0.68945531, -0.6339549, -0.64779226, -0.72921559, -0.75137744, -0.73587286, -0.72468758, -0.75455887, -0.6949301, -0.66419364, -0.78141906, -0.71708496, -0.74957072, -0.75440543, -0.79022752, -0.81582876, -0.85003708, -0.79718986, -0.70908029, -0.7948793, -0.82351793, -0.82099982, -0.90962242, -0.82940291, -0.82645972, -0.88457099, -0.90277854, -0.73435763, -0.89281041, -0.8731476, -0.90199506, -0.87104215, -0.93992167, -0.88914756, -0.90782778, -0.87556893, -0.89981662, -0.76902729, -0.83687477, -0.93247417, -0.86291953, -0.85195962, -0.81303577, -0.93169424, -0.88172655, -1.07267545, -0.97001875, -1.00105324, -1.00428899, -0.98393847, -1.03255942, -0.92122492, -1.07395808, -1.0128527, -1.05137684, -1.047103, -1.07584361, -1.07115095, -1.18445538, -1.07431948, -0.99711779, -1.05784667, -1.10645181, -1.12273395, -1.10840479, -1.15898328, -1.20715507, -1.14028285, -1.20342827, -1.24761428, -1.22032985, -1.27974244, -1.22850816, -1.26746488, -1.33153367, -1.14839422, -1.18404104, -1.23199741, -1.32498703, -1.26100096, -1.24243304, -1.2737479, -1.28610737, -1.30884853, -1.24839463, -1.16597388, -1.24925546, -1.16761645, -1.19659387, -1.21711949, -1.24061676, -1.26013109, -1.11073331, -1.22445389, -1.33253102, -1.20538906, -1.28740177, -1.38325577, -1.11760803, -1.28938927, -1.28976635, -1.36248042, -1.34015072, -1.31408804, -1.21046288, -1.25856053, -1.26922239, -1.15383794, -1.205826, -1.26086174, -1.23678076, -1.31317363, -1.37652076, -1.41586408, -1.20597583, -1.36710643, -1.34255233, -1.25131453, -1.2870645, -1.33174301, -1.40020549, -1.30694795, -1.2045447, -1.28020176, -1.42512079, -1.34800498, -1.42910301, -1.42657412, -1.40040383, -1.44534752, -1.31612798, -1.31328765, -1.2645929, -1.31730589, -1.44917086, -1.48042685, -1.48246777, -1.6069132, -1.49147634, -1.59657146, -1.49438681, -1.53218087, -1.61774453, -1.49481865, -1.46159514, -1.48785503, -1.59432746, -1.62819133, -1.71381539, -1.68348601, -1.7161616, -1.67665743, -1.68295333, -1.65154049, -1.52324358, -1.57369266, -1.5682697, -1.62700899, -1.71863545, -1.70241582, -1.75268931, -1.59710926, -1.66789895, -1.81990938, -1.72930759, -1.81298228, -1.74055081, -1.61731119, -1.73926896, -1.85620289, -1.73819272, -1.81750964, -1.82375387, -1.89273653, -1.88659901, -1.83943754, -1.79818326, -1.88636852, -1.69756045, -1.71421935, -1.87550076, -1.95622633, -1.83663434, -1.91914803, -1.91554095, -1.95163205, -1.89719334, -2.00565679, -1.88185899, -2.01510661, -2.02584106, -2.04327536, -2.00180772, -2.04674097, -1.96989144, -1.96809263, -2.05356691, -2.02755143, -2.04031214, -2.06345679, -2.05680446, -2.05412966, -2.07028399, -2.13129749, -2.19773722, -2.14798477, -2.02987559, -2.19712272, -2.12220486, -2.10896356, -2.17962118, -2.17513158, -2.16685523, -2.21700219, -2.10393398, -2.13717561, -2.2089672, -2.16493494, -2.18153417, -2.34229158, -2.16215572, -2.25785433, -2.22596349, -2.25187127, -2.35730309, -2.27379377, -2.32334743, -2.29175604, -2.20314771, -2.34439824, -2.38119664, -2.29790384, -2.40038917, -2.27058666, -2.40768479, -2.4473483, -2.60870625, -2.54751462, -2.53021285, -2.5877664, -2.41339714, -2.50834546, -2.61013394, -2.33705979, -2.54412908, -2.37872198, -2.32201169, -2.49044799, -2.48988715, -2.52837286, -2.4771429, -2.41691251, -2.41615598, -2.54943333, -2.44480101, -2.53825643, -2.40334417, -2.36938469, -2.37232876, -2.38218338, -2.4007207, -2.448537, -2.40978314, -2.50198391, -2.58420146, -2.48682817, -2.48172298, -2.45436571, -2.4967308, -2.43939981, -2.58457166, -2.43048312, -2.56066294, -2.45549519, -2.47804837, -2.42841964, -2.51133231, -2.44386246, -2.60310665, -2.67063121, -2.62883095, -2.64996527, -2.65067169, -2.71624159, -2.59601593, -2.74491664, -2.758366, -2.66158956, -2.63083217, -2.8731213, -2.8308766, -2.8027204, -2.7521968, -2.82272042, -2.8164733, -2.88768866, -2.90256896, -2.84367916, -2.9228607, -3.07481535, -2.88676048, -3.02662656, -2.95227409, -2.9718118, -2.96904895, -2.92507519, -2.90994016, -3.03592661, -2.86042929, -2.93424849, -2.86955675, -2.91288022, -2.92450324, -2.99792798, -3.05979151, -3.03700993, -2.93710315, -3.06990026, -2.98513574, -3.00533434, -2.97877259, -3.02315398, -3.08308014, -3.10903297, -3.15263997, -3.02982441, -3.26555892, -3.13993419, -3.41825506, -3.19378873, -3.23176941, -3.34563346, -3.29244211, -3.32094009, -3.41552083, -3.50898568, -3.28387452, -3.50556782, -3.49307458, -3.55551364, -3.45119325, -3.49144363, -3.35562487, -3.3305146, -3.49546844, -3.43299379, -3.43079581, -3.48817712, -3.52600011, -3.41451394, -3.45294882, -3.47961549, -3.50905251, -3.50087667, -3.62196941, -3.64036995, -3.66396678, -3.78242859, -3.8272262, -3.94477002, -3.94973945, -3.80467535, -3.85042978, -3.72641937, -3.77263417, -3.66180042, -3.91142471, -3.87559929, -3.81638351, -3.91497848, -3.9541892, -3.92320042, -3.99715778, -4.08213121, -4.02036058, -4.06936996, -3.94495614, -4.09507289, -4.03485348, -4.12562065, -4.23981777, -4.10507388, -4.21910866, -4.12512183, -4.28665132, -4.31376275, -4.18817295, -4.33383404, -4.36005697, -4.26141923, -4.18360141, -4.24917635, -4.35052763, -4.33966549, -4.38850899, -4.40321474, -4.49714659, -4.50771025, -4.51335601, -4.57639867, -4.42819556, -4.556029, -4.53683211, -4.47300718, -4.55151022, -4.67492457, -4.75698858, -4.63938981, -4.58238998, -4.66015878, -4.55188925, -4.6985391, -4.57481399], 9 "Offset Applied?":bool=TRUE) -> (14 "Save Array out":string[][](array[string]), 17 "Full Array":string[][](array[string]), 19 "Canceled":bool)   [LabVIEW 2024]
uses:
  DataCluster_TCAL.ctl
  <vilib>/vision/Image Controls.llb/IMAQ Image.ctl
  TCE_Config.ctl
panel:
  in  "Nm(T)":bool
  in  "SaveFrozen":bool=TRUE caption="Frozen Fraction"
  in  "SaveMelt":bool=TRUE caption="Melting Point"
  in  "SaveFreeze":bool=TRUE caption="Freezing Point"
  in  "SaveTemp":bool=TRUE caption="Temperatures"
  out "Data Array":string[][](array[string])
  in  "Cancel":bool
  in  "OK":bool
  # "Settings"
  # "File Preview"
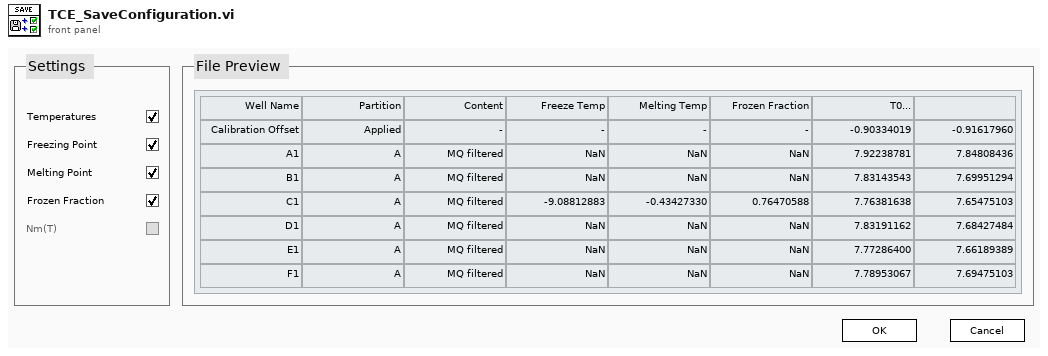
[diagram p1: front panel]
types:
  T1 = typedef "DataCluster_TCAL.ctl" = cluster{"Core":cluster{"Current VI Reference":refnum<vi>, "Close Panel on Exit?":bool}, "Image Out":T2, "State":i32, "Points":cluster{"Top Left":T3, "Top Right":T3, "Bottom Left":T3, "Bottom Right":T3, "x space 2":dbl, "y space 2":sgl, "x_space":sgl, "y_space":sgl, "Pixels":cluster{"X":i32, "Y":i32}[][], "Fixpoint":T3}, "img_array":T2[], "Temps":dbl[], "Temps_Array":dbl[][], "Scan Area":dbl, "Fixpoint Area":dbl, "Config":T4, "PCR Size":u16, "ImageCount":i32, "ShowGradient":bool}
  T2 = typedef "IMAQ Image.ctl" = refnum<image>
  T3 = typedef "IMAQ Point" = cluster{"X":sgl, "Y":sgl}
  T4 = typedef "TCE_Config.ctl" = cluster{"Freezing":cluster{"Cutoff":dbl, "EndIndex":i32}}
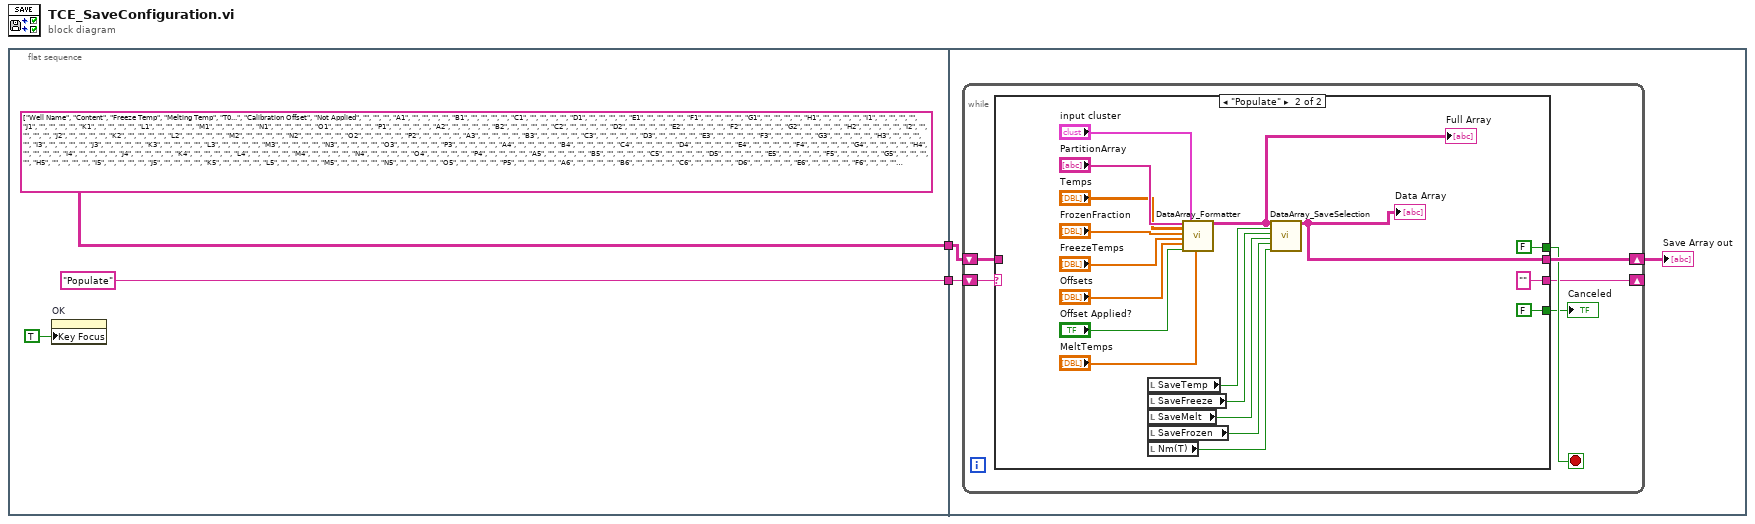
[diagram p0: block diagram]
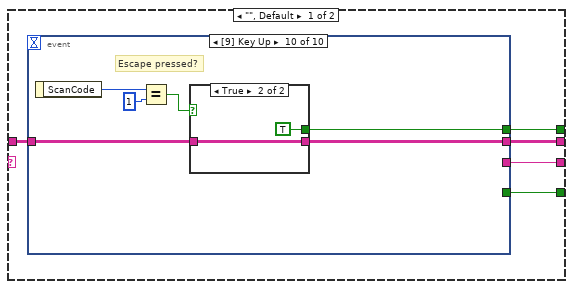
[diagram p2: hidden frame]
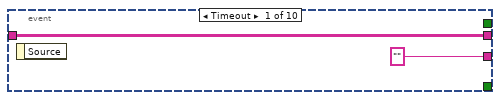
[diagram p3: hidden frame]
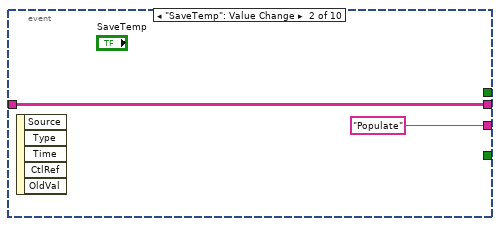
[diagram p4: hidden frame]
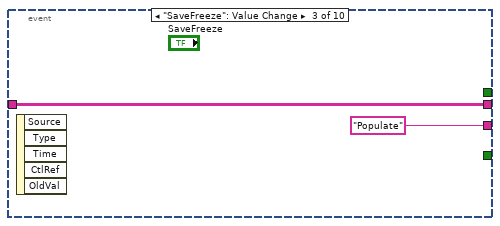
[diagram p5: hidden frame]
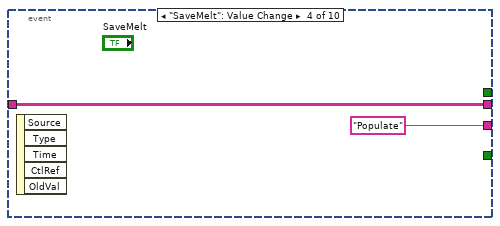
[diagram p6: hidden frame]
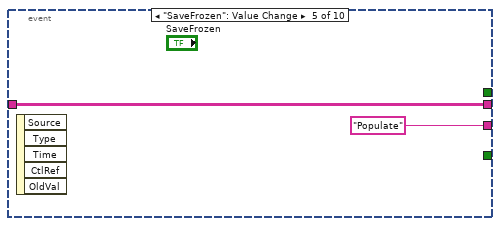
[diagram p7: hidden frame]
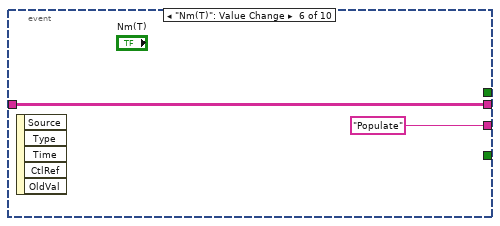
[diagram p8: hidden frame]
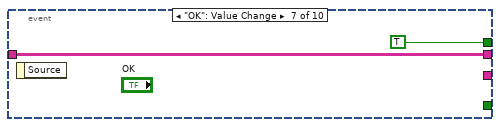
[diagram p9: hidden frame]
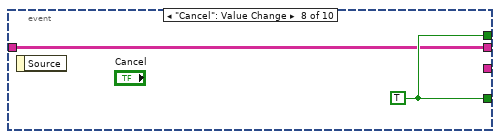
[diagram p10: hidden frame]
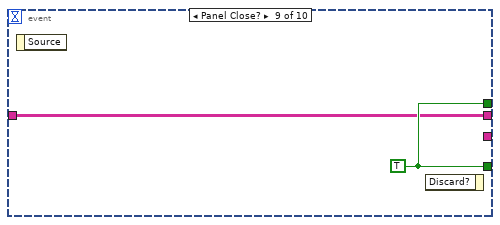
[diagram p11: hidden frame]
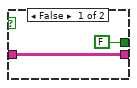
[diagram p12: hidden frame]
diagram:
  n1 = flat-sequence {
    tunnel: [string[][] [["Well Name", "Content", "Freeze Temp", "Melting Temp", "T0..."], ["Calibration Offset", "Not Applied", "", "", ""], ["A1", "", "", "", ""], ["B1", "", "", "", ""], ["C1", "", "", "", ""], ["D1", "", "", "", ""], ["E1", "", "", "", ""], ["F1", "", "", "", ""], ["G1", "", "", "", ""], ["H1", "", "", "", ""], ["I1", "", "", "", ""], ["J1", "", "", "", ""], ["K1", "", "", "", ""], ["L1", "", "", "", ""], ["M1", "", "", "", ""], ["N1", "", "", "", ""], ["O1", "", "", "", ""], ["P1", "", "", "", ""], ["A2", "", "", "", ""], ["B2", "", "", "", ""], ["C2", "", "", "", ""], ["D2", "", "", "", ""], ["E2", "", "", "", ""], ["F2", "", "", "", ""], ["G2", "", "", "", ""], ["H2", "", "", "", ""], ["I2", "", "", "", ""], ["J2", "", "", "", ""], ["K2", "", "", "", ""], ["L2", "", "", "", ""], ["M2", "", "", "", ""], ["N2", "", "", "", ""], ["O2", "", "", "", ""], ["P2", "", "", "", ""], ["A3", "", "", "", ""], ["B3", "", "", "", ""], ["C3", "", "", "", ""], ["D3", "", "", "", ""], ["E3", "", "", "", ""], ["F3", "", "", "", ""], ["G3", "", "", "", ""], ["H3", "", "", "", ""], ["I3", "", "", "", ""], ["J3", "", "", "", ""], ["K3", "", "", "", ""], ["L3", "", "", "", ""], ["M3", "", "", "", ""], ["N3", "", "", "", ""], ["O3", "", "", "", ""], ["P3", "", "", "", ""], ["A4", "", "", "", ""], ["B4", "", "", "", ""], ["C4", "", "", "", ""], ["D4", "", "", "", ""], ["E4", "", "", "", ""], ["F4", "", "", "", ""], ["G4", "", "", "", ""], ["H4", "", "", "", ""], ["I4", "", "", "", ""], ["J4", "", "", "", ""], ["K4", "", "", "", ""], ["L4", "", "", "", ""], ["M4", "", "", "", ""], ["N4", "", "", "", ""], ["O4", "", "", "", ""], ["P4", "", "", "", ""], ["A5", "", "", "", ""], ["B5", "", "", "", ""], ["C5", "", "", "", ""], ["D5", "", "", "", ""], ["E5", "", "", "", ""], ["F5", "", "", "", ""], ["G5", "", "", "", ""], ["H5", "", "", "", ""], ["I5", "", "", "", ""], ["J5", "", "", "", ""], ["K5", "", "", "", ""], ["L5", "", "", "", ""], ["M5", "", "", "", ""], ["N5", "", "", "", ""], ["O5", "", "", "", ""], ["P5", "", "", "", ""], ["A6", "", "", "", ""], ["B6", "", "", "", ""], ["C6", "", "", "", ""], ["D6", "", "", "", ""], ["E6", "", "", "", ""], ["F6", "", "", "", ""], ["G6", "", "", "", ""], ["H6", "", "", "", ""], ["I6", "", "", "", ""], ["J6", "", "", "", ""], ["K6", "", "", "", ""], ["L6", "", "", "", ""], ["M6", "", "", "", ""], ["N6", "", "", "", ""], ["O6", "", "", "", ""], ["P6", "", "", "", ""], ["A7", "", "", "", ""], ["B7", "", "", "", ""], ["C7", "", "", "", ""], ["D7", "", "", "", ""], ["E7", "", "", "", ""], ["F7", "", "", "", ""], ["G7", "", "", "", ""], ["H7", "", "", "", ""], ["I7", "", "", "", ""], ["J7", "", "", "", ""], ["K7", "", "", "", ""], ["L7", "", "", "", ""], ["M7", "", "", "", ""], ["N7", "", "", "", ""], ["O7", "", "", "", ""], ["P7", "", "", "", ""], ["A8", "", "", "", ""], ["B8", "", "", "", ""], ["C8", "", "", "", ""], ["D8", "", "", "", ""], ["E8", "", "", "", ""], ["F8", "", "", "", ""], ["G8", "", "", "", ""], ["H8", "", "", "", ""], ["I8", "", "", "", ""], ["J8", "", "", "", ""], ["K8", "", "", "", ""], ["L8", "", "", "", ""], ["M8", "", "", "", ""], ["N8", "", "", "", ""], ["O8", "", "", "", ""], ["P8", "", "", "", ""], ["A9", "", "", "", ""], ["B9", "", "", "", ""], ["C9", "", "", "", ""], ["D9", "", "", "", ""], ["E9", "", "", "", ""], ["F9", "", "", "", ""], ["G9", "", "", "", ""], ["H9", "", "", "", ""], ["I9", "", "", "", ""], ["J9", "", "", "", ""], ["K9", "", "", "", ""], ["L9", "", "", "", ""], ["M9", "", "", "", ""], ["N9", "", "", "", ""], ["O9", "", "", "", ""], ["P9", "", "", "", ""], ["A10", "", "", "", ""], ["B10", "", "", "", ""], ["C10", "", "", "", ""], ["D10", "", "", "", ""], ["E10", "", "", "", ""], ["F10", "", "", "", ""], ["G10", "", "", "", ""], ["H10", "", "", "", ""], ["I10", "", "", "", ""], ["J10", "", "", "", ""], ["K10", "", "", "", ""], ["L10", "", "", "", ""], ["M10", "", "", "", ""], ["N10", "", "", "", ""], ["O10", "", "", "", ""], ["P10", "", "", "", ""], ["A11", "", "", "", ""], ["B11", "", "", "", ""], ["C11", "", "", "", ""], ["D11", "", "", "", ""], ["E11", "", "", "", ""], ["F11", "", "", "", ""], ["G11", "", "", "", ""], ["H11", "", "", "", ""], ["I11", "", "", "", ""], ["J11", "", "", "", ""], ["K11", "", "", "", ""], ["L11", "", "", "", ""], ["M11", "", "", "", ""], ["N11", "", "", "", ""], ["O11", "", "", "", ""], ["P11", "", "", "", ""], ["A12", "", "", "", ""], ["B12", "", "", "", ""], ["C12", "", "", "", ""], ["D12", "", "", "", ""], ["E12", "", "", "", ""], ["F12", "", "", "", ""], ["G12", "", "", "", ""], ["H12", "", "", "", ""], ["I12", "", "", "", ""], ["J12", "", "", "", ""], ["K12", "", "", "", ""], ["L12", "", "", "", ""], ["M12", "", "", "", ""], ["N12", "", "", "", ""], ["O12", "", "", "", ""], ["P12", "", "", "", ""], ["A13", "", "", "", ""], ["B13", "", "", "", ""], ["C13", "", "", "", ""], ["D13", "", "", "", ""], ["E13", "", "", "", ""], ["F13", "", "", "", ""], ["G13", "", "", "", ""], ["H13", "", "", "", ""], ["I13", "", "", "", ""], ["J13", "", "", "", ""], ["K13", "", "", "", ""], ["L13", "", "", "", ""], ["M13", "", "", "", ""], ["N13", "", "", "", ""], ["O13", "", "", "", ""], ["P13", "", "", "", ""], ["A14", "", "", "", ""], ["B14", "", "", "", ""], ["C14", "", "", "", ""], ["D14", "", "", "", ""], ["E14", "", "", "", ""], ["F14", "", "", "", ""], ["G14", "", "", "", ""], ["H14", "", "", "", ""], ["I14", "", "", "", ""], ["J14", "", "", "", ""], ["K14", "", "", "", ""], ["L14", "", "", "", ""], ["M14", "", "", "", ""], ["N14", "", "", "", ""], ["O14", "", "", "", ""], ["P14", "", "", "", ""], ["A15", "", "", "", ""], ["B15", "", "", "", ""], ["C15", "", "", "", ""], ["D15", "", "", "", ""], ["E15", "", "", "", ""], ["F15", "", "", "", ""], ["G15", "", "", "", ""], ["H15", "", "", "", ""], ["I15", "", "", "", ""], ["J15", "", "", "", ""], ["K15", "", "", "", ""], ["L15", "", "", "", ""], ["M15", "", "", "", ""], ["N15", "", "", "", ""], ["O15", "", "", "", ""], ["P15", "", "", "", ""], ["A16", "", "", "", ""], ["B16", "", "", "", ""], ["C16", "", "", "", ""], ["D16", "", "", "", ""], ["E16", "", "", "", ""], ["F16", "", "", "", ""], ["G16", "", "", "", ""], ["H16", "", "", "", ""], ["I16", "", "", "", ""], ["J16", "", "", "", ""], ["K16", "", "", "", ""], ["L16", "", "", "", ""], ["M16", "", "", "", ""], ["N16", "", "", "", ""], ["O16", "", "", "", ""], ["P16", "", "", "", ""], ["A17", "", "", "", ""], ["B17", "", "", "", ""], ["C17", "", "", "", ""], ["D17", "", "", "", ""], ["E17", "", "", "", ""], ["F17", "", "", "", ""], ["G17", "", "", "", ""], ["H17", "", "", "", ""], ["I17", "", "", "", ""], ["J17", "", "", "", ""], ["K17", "", "", "", ""], ["L17", "", "", "", ""], ["M17", "", "", "", ""], ["N17", "", "", "", ""], ["O17", "", "", "", ""], ["P17", "", "", "", ""], ["A18", "", "", "", ""], ["B18", "", "", "", ""], ["C18", "", "", "", ""], ["D18", "", "", "", ""], ["E18", "", "", "", ""], ["F18", "", "", "", ""], ["G18", "", "", "", ""], ["H18", "", "", "", ""], ["I18", "", "", "", ""], ["J18", "", "", "", ""], ["K18", "", "", "", ""], ["L18", "", "", "", ""], ["M18", "", "", "", ""], ["N18", "", "", "", ""], ["O18", "", "", "", ""], ["P18", "", "", "", ""], ["A19", "", "", "", ""], ["B19", "", "", "", ""], ["C19", "", "", "", ""], ["D19", "", "", "", ""], ["E19", "", "", "", ""], ["F19", "", "", "", ""], ["G19", "", "", "", ""], ["H19", "", "", "", ""], ["I19", "", "", "", ""], ["J19", "", "", "", ""], ["K19", "", "", "", ""], ["L19", "", "", "", ""], ["M19", "", "", "", ""], ["N19", "", "", "", ""], ["O19", "", "", "", ""], ["P19", "", "", "", ""], ["A20", "", "", "", ""], ["B20", "", "", "", ""], ["C20", "", "", "", ""], ["D20", "", "", "", ""], ["E20", "", "", "", ""], ["F20", "", "", "", ""], ["G20", "", "", "", ""], ["H20", "", "", "", ""], ["I20", "", "", "", ""], ["J20", "", "", "", ""], ["K20", "", "", "", ""], ["L20", "", "", "", ""], ["M20", "", "", "", ""], ["N20", "", "", "", ""], ["O20", "", "", "", ""], ["P20", "", "", "", ""], ["A21", "", "", "", ""], ["B21", "", "", "", ""], ["C21", "", "", "", ""], ["D21", "", "", "", ""], ["E21", "", "", "", ""], ["F21", "", "", "", ""], ["G21", "", "", "", ""], ["H21", "", "", "", ""], ["I21", "", "", "", ""], ["J21", "", "", "", ""], ["K21", "", "", "", ""], ["L21", "", "", "", ""], ["M21", "", "", "", ""], ["N21", "", "", "", ""], ["O21", "", "", "", ""], ["P21", "", "", "", ""], ["A22", "", "", "", ""], ["B22", "", "", "", ""], ["C22", "", "", "", ""], ["D22", "", "", "", ""], ["E22", "", "", "", ""], ["F22", "", "", "", ""], ["G22", "", "", "", ""], ["H22", "", "", "", ""], ["I22", "", "", "", ""], ["J22", "", "", "", ""], ["K22", "", "", "", ""], ["L22", "", "", "", ""], ["M22", "", "", "", ""], ["N22", "", "", "", ""], ["O22", "", "", "", ""], ["P22", "", "", "", ""], ["A23", "", "", "", ""], ["B23", "", "", "", ""], ["C23", "", "", "", ""], ["D23", "", "", "", ""], ["E23", "", "", "", ""], ["F23", "", "", "", ""], ["G23", "", "", "", ""], ["H23", "", "", "", ""], ["I23", "", "", "", ""], ["J23", "", "", "", ""], ["K23", "", "", "", ""], ["L23", "", "", "", ""], ["M23", "", "", "", ""], ["N23", "", "", "", ""], ["O23", "", "", "", ""], ["P23", "", "", "", ""], ["A24", "", "", "", ""], ["B24", "", "", "", ""], ["C24", "", "", "", ""], ["D24", "", "", "", ""], ["E24", "", "", "", ""], ["F24", "", "", "", ""], ["G24", "", "", "", ""], ["H24", "", "", "", ""], ["I24", "", "", "", ""], ["J24", "", "", "", ""], ["K24", "", "", "", ""], ["L24", "", "", "", ""], ["M24", "", "", "", ""], ["N24", "", "", "", ""], ["O24", "", "", "", ""], ["P24", "", "", "", ""]] ("Data Array out")] -> w2
    tunnel: ["Populate"] -> w1
    tunnel: w2 -> [w8]
    tunnel: w1 -> [w7]
    frame #0 {
      n2 = property on="OK" class="Bool"("Key Focus"=TRUE) -> ()  [unwired: 2 in, 2 out]
    }
    frame #1 {
      n3 = while {
        shift-right: [w14] -> w6
        shift-left: w8 -> [w13]
        shift-right: [w9] -> _
        shift-left: w7 -> [w10]
        stop <- w12 stop-if-true
        n4 = case shown="\"Populate\"" w10 {
          tunnel: [w19 w48] -> w14
          tunnel: w13 -> [w18 _]
          tunnel: [w17 FALSE] -> w12
          tunnel: [w16 FALSE] -> w11
          tunnel: [w15 ""] -> w9
          frame "", Default {
            n5 = event shown="[9] Key Up" {
              selector: _ -> [_ _ _ _ _ _ _ _ _ _]
              dyn-events: _ -> [_ _ _ _ _ _ _ _ _ _]
              timeout: _ -> [_ _ _ _ _ _ _ _ _ _]
              tunnel: w18 -> [w20 w22 w24 w26 w28 w30 w33 w34 w36 w38]
              tunnel: [w20 w22 w24 w26 w28 w30 w33 w34 w36 w39] -> w19
              tunnel: [_ _ _ _ _ _ TRUE w35 w37 w43] -> w17
              tunnel: [_ _ _ _ _ _ _ w35 w37 _] -> w16
              tunnel: ["" "Populate" "Populate" "Populate" "Populate" "Populate" _ _ _ _] -> w15
              event Timeout {
                n6 = event-data() -> ()  [unwired: 1 in, 1 out]
              }
              event "SaveTemp": Value Change {
                n7 = event-data() -> ()  [unwired: 1 in, 5 out]
              }
              event "SaveFreeze": Value Change {
                n8 = event-data() -> ()  [unwired: 1 in, 5 out]
              }
              event "SaveMelt": Value Change {
                n9 = event-data() -> ()  [unwired: 1 in, 5 out]
              }
              event "SaveFrozen": Value Change {
                n10 = event-data() -> ()  [unwired: 1 in, 5 out]
              }
              event "Nm(T)": Value Change {
                n11 = event-data() -> ()  [unwired: 1 in, 5 out]
              }
              event "OK": Value Change {
                n12 = event-data() -> ()  [unwired: 1 in, 1 out]
              }
              event "Cancel": Value Change {
                w35 = TRUE
                n13 = event-data() -> ()  [unwired: 1 in, 1 out]
              }
              event Panel Close? {
                w37 = TRUE
                n14 = event-data() -> ()  [unwired: 1 in, 1 out]
                n15 = event-data() -> ()  [unwired: 2 in, 1 out]
              }
              event Key Up {
                # "Escape pressed?"
                n16 = event-data() -> ("ScanCode"=w42:i16)  [unwired: 1 in]
                n17 = Equal?(x=w42, y=i16 1) -> (x = y?=w40:bool)
                n18 = case shown="True" w40 {
                  tunnel: [FALSE TRUE] -> w43
                  tunnel: [w45 w46] -> w39
                  tunnel: w38 -> [w45 w46]
                  frame False {
                  }
                  frame True {
                  }
                }
              }
            }
          }
          frame "Populate" {
            n19 = local read "SaveTemp"() -> (w61:bool)
            n20 = local read "SaveFreeze"() -> (w57:bool)
            n21 = local read "SaveMelt"() -> (w58:bool)
            n22 = local read "SaveFrozen"() -> (w59:bool)
            n23 = local read "Nm(T)"() -> (w60:bool)
            n24 = call "DataArray_Formatter.vi"("PartitionArray"="PartitionArray", "Temps"="Temps", "FrozenFraction"="FrozenFraction", "FreezeTemps"="FreezeTemps", "Offsets"="Offsets", "Offset Applied?"="Offset Applied?", "input cluster"="input cluster", "MeltTemps"="MeltTemps") -> ("Data Array"=w62:string[][])  [unwired: 11 in]
            "Full Array" <- w62
            n25 = call "DataArray_SaveSelection.vi"("Data Array"=w62, "SaveTemp"=w61, "SaveFreeze"=w57, "SaveMelt"=w58, "SaveFrozen"=w59, "Nm(T)"=w60) -> ("Data Array out"=w48:string[][])  [unwired: 13 in]
            "Data Array" <- w48
          }
        }
        "Canceled" <- w11
      }
      "Save Array out" <- w6
    }
  }
